vi "Find USB Device Name_v3.vi"() -> ()   [LabVIEW 2016]
panel:
  out "Roboteq":refnum<visa-resource-name>
  in  "Keyword for Roboteq":string
  out "List of card in the Computer 2":string[](array[string])
  out "Interface Information:Interface Description 2":string
  out "General Settings:Resource Name 2":string
  out "Uno":refnum<visa-resource-name>
  in  "Keyword for Uno":string
  out "List of card in the Computer":string[](array[string])
  out "Interface Information:Interface Description":string
  out "General Settings:Resource Name":string
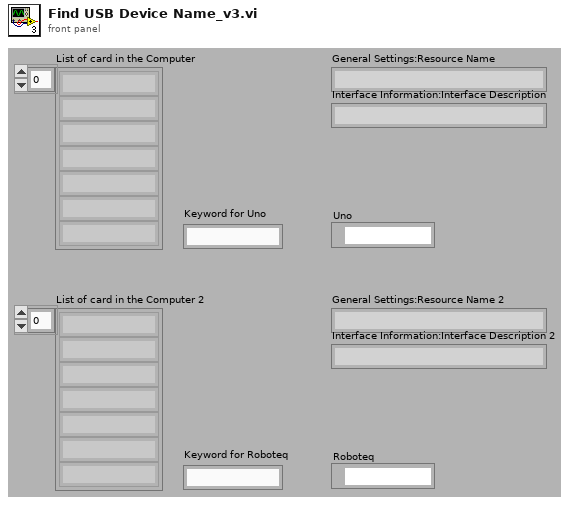
[diagram p1: front panel]
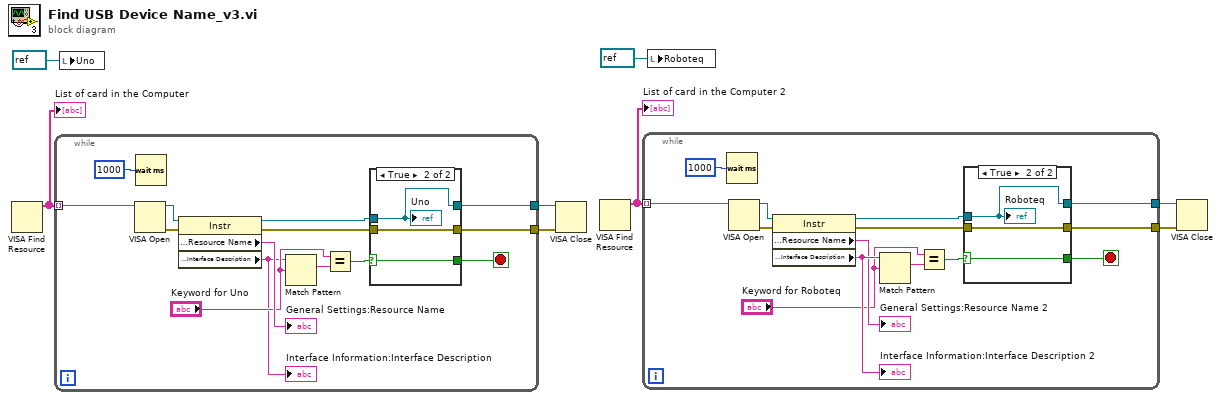
[diagram p0: block diagram]
diagram:
  n1 = VISA Find Resource() -> (3:w8:string[])  [unwired: 3 in, 2 out]
  "List of card in the Computer" <- w8
  n2 = while {
    tunnel: w8 -> [w19] mode=indexing
    tunnel: [w11] -> w4
    tunnel: [w9] -> w3
    stop <- w12 stop-if-true
    n3 = VISA Open(VISA resource name=w19) -> (VISA resource name=w21:refnum<visa-resource-name>, error out=w22:errorcluster)  [unwired: 4 in]
    n4 = Wait (ms)(milliseconds to wait=1000) -> ()  [unwired: 1 out]
    n5 = property class="Instr"(reference=w21, error in=w22) -> (reference out=w17:refnum<visa-resource-name>, error out=w10:errorcluster, "General Settings:Resource Name"=→"General Settings:Resource Name":string, "Interface Information:Interface Description"=w13:string)
    "Interface Information:Interface Description" <- w13
    n6 = Match Pattern(string=w13, regular expression="Keyword for Uno") -> (match substring=w15:string)  [unwired: 1 in, 3 out]
    n7 = Equal?(x="Keyword for Uno", y=w15) -> (x = y?=w16:bool)
    n8 = case shown="True" w16 {
      selector: w16 -> [_ w25]
      tunnel: w17 -> [_ w23]
      tunnel: [_ w25] -> w12
      tunnel: [_ w24] -> w11
      tunnel: w10 -> [_ w24]
      tunnel: [_ w23] -> w9
      frame False {
      }
      frame True {
        "Uno" <- w23
      }
    }
  }
  n9 = local write "Uno"(refnum<visa-resource-name> refnum ("Uno")) -> ()
  n10 = VISA Close(VISA resource name=w3, error in (no error)=w4) -> ()  [unwired: 1 out]
  n11 = VISA Find Resource() -> (3:w6:string[])  [unwired: 3 in, 2 out]
  "List of card in the Computer 2" <- w6
  n12 = while {
    tunnel: w6 -> [w37] mode=indexing
    tunnel: [w28] -> w2
    tunnel: [w26] -> w1
    stop <- w29 stop-if-true
    n13 = Wait (ms)(milliseconds to wait=1000) -> ()  [unwired: 1 out]
    n14 = VISA Open(VISA resource name=w37) -> (VISA resource name=w38:refnum<visa-resource-name>, error out=w39:errorcluster)  [unwired: 4 in]
    n15 = property class="Instr"(reference=w38, error in=w39) -> (reference out=w35:refnum<visa-resource-name>, error out=w27:errorcluster, "General Settings:Resource Name"=→"General Settings:Resource Name 2":string, "Interface Information:Interface Description"=w32:string)
    "Interface Information:Interface Description 2" <- w32
    n16 = Match Pattern(string=w32, regular expression="Keyword for Roboteq") -> (match substring=w33:string)  [unwired: 1 in, 3 out]
    n17 = Equal?(x="Keyword for Roboteq", y=w33) -> (x = y?=w34:bool)
    n18 = case shown="True" w34 {
      selector: w34 -> [_ w42]
      tunnel: w35 -> [_ w40]
      tunnel: [_ w42] -> w29
      tunnel: [_ w41] -> w28
      tunnel: w27 -> [_ w41]
      tunnel: [_ w40] -> w26
      frame False {
      }
      frame True {
        "Roboteq" <- w40
      }
    }
  }
  n19 = local write "Roboteq"(refnum<visa-resource-name> refnum ("Roboteq")) -> ()
  n20 = VISA Close(VISA resource name=w1, error in (no error)=w2) -> ()  [unwired: 1 out]
